vi "SetTimeout.vi"(8 "error in (no error)":errorcluster, 10 "Numeric":dbl, 11 "Point Grey Camera in":refnum<class "Point Grey Camera.lvclass">) -> (0 "error out":errorcluster, 3 "Point Grey Camera out":refnum<class "Point Grey Camera.lvclass">)   [LabVIEW 2020, in "Point Grey Camera.lvclass"]
uses:
  Point Grey Camera.lvclass
  Point Grey Camera.lvclass/Point Grey Camera.ctl
  <resource>/objmgr/imaqdx.rc
  NI_Vision_Acquisition_Software.lvlib
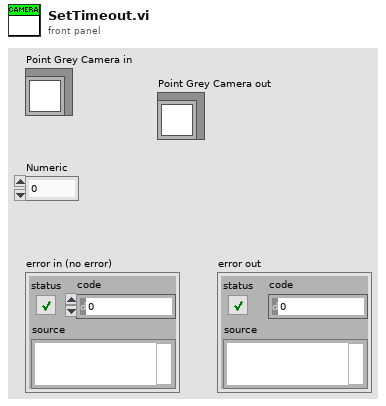
[diagram p1: front panel]
types:
  T1 = typedef "IMAQdx.ctl" = refnum<k21>
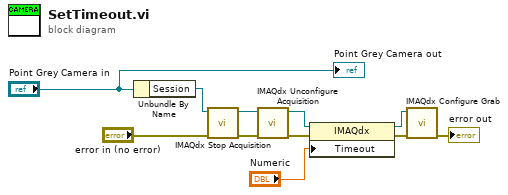
[diagram p0: block diagram]
diagram:
  n1 = Unbundle By Name("Point Grey Camera in") -> ("Session"=w11:T1)
  n2 = call "IMAQdx Stop Acquisition.vi"("error in"="error in (no error)", "Session In"=w11) -> ("error out"=w6:errorcluster, "Session Out"=w3:T1)  [unwired: 8 out]
  n3 = call "IMAQdx Unconfigure Acquisition.vi"("error in"=w6, "Session In"=w3) -> ("error out"=w7:errorcluster, "Session Out"=w4:T1)  [unwired: 8 out]
  n4 = property class="IMAQdx"(reference=w4, error in=w7, "Timeout"="Numeric") -> (reference out=w5:T1, error out=w9:errorcluster)
  n5 = call "IMAQdx Configure Grab.vi"("error in"=w9, "Session In"=w5) -> ("error out"=→"error out":errorcluster)  [unwired: 1 in, 8 out]
  "Point Grey Camera out" <- "Point Grey Camera in"
